vi "Parse ASCII Data.vi"(2 "ASCII Data (Empty)":string) -> (15 "Measurement":dbl, 16 "Channel":i32, 17 "Units":string)   [LabVIEW 2009, in "Keithley 2000.lvlib"]
doc: "This VI parses the ASCII data returned by the instrument and returns the measurement value, the units, and the channel number.\n\nThe input ASCII data should be in this format (the format returned by the instrument):\n±1.23456789E±00VDC, 0INTCHAN"
uses:
  Keithley 2000/Keithley 2000.lvlib
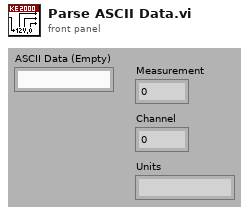
[diagram p1: front panel]
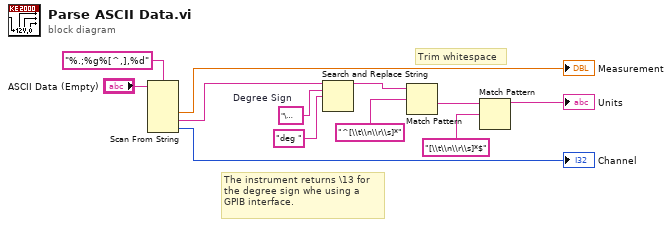
[diagram p0: block diagram]
diagram:
  w11 = "\u0013"  # Degree Sign
  # "Trim whitespace"
  # "The instrument returns \\13 for\nthe degree sign whe using a\nGPIB interface."
  n1 = Scan From String(format string="%.;%g%[^,],%d", input string="ASCII Data (Empty)") -> (output 1=→"Measurement":dbl, output 2=w10:string, output 3=→"Channel":i32)  [unwired: 5 in, 3 out]
  n2 = Search and Replace String(input string=w10, search string=w11, replace string="deg " ("replace string (\"\")")) -> (result string=w2:string)  [unwired: 5 in, 3 out]
  n3 = Match Pattern(string=w2, regular expression="^[\\t\\n\\r\\s]*") -> (after substring=w5:string)  [unwired: 1 in, 3 out]
  n4 = Match Pattern(string=w5, regular expression="[\\t\\n\\r\\s]*$") -> (before substring=→"Units":string)  [unwired: 1 in, 3 out]
